vi "Read ECAT VARs.vi"(7 "R/W Case":T7, 8 "error in (no error)":errorcluster, 9 "Output FIFO buffer in":dbl[](array[numeric]), 10 "I/O Input Data in":T1 {"BD Refs"."Data Reference" format="%.0x"}, 11 "I/O Output Vars in":T4[](array[typedef]) {"VS ref" format="%.0x"}) -> (0 "error out":errorcluster, 1 "Output FIFO buffer out":dbl[](array[numeric]), 2 "I/O Input Data out":T1 {"BD Refs"."Data Reference" format="%.0x"}, 3 "I/O Output Vars out":T4[](array[typedef]) {"VS ref" format="%.0x"})   [LabVIEW 2020, in "SEECD Engine.lvlib"]
uses:
  SEECD Engine.lvlib
  Type Defs/RW Case.ctl
  Type Defs/Generic ECAT Slave IOV Cluster.ctl
  <vilib>/NI VeriStand/Custom Device API/Custom Device Item Ref.ctl
  Shared/Type Defs/UDV Data Type.ctl
  Type Defs/Input Data.ctl
  <vilib>/NI VeriStand/Custom Device API/Block Data Reference.ctl
  <vilib>/NI VeriStand/Custom Device API/Data Reference.ctl
  <vilib>/NI VeriStand/Custom Device API/Global Data Refs.vi
  <vilib>/NI VeriStand/Custom Device API/Custom Device API.lvlib
  <vilib>/NI VeriStand/Custom Device Tools/Custom Device Utility Library/Custom Device Utility Library.lvlib
  Shared/SEECD Shared.lvlib
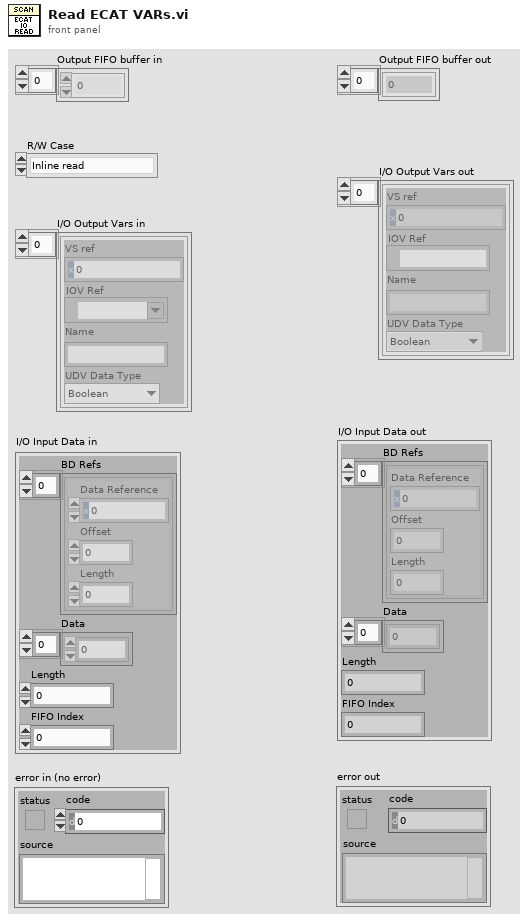
[diagram p1: front panel]
types:
  T1 = typedef "SEECD Engine.lvlib/Input Data.ctl" = cluster{"BD Refs":T2[], "Data":dbl[], "Length":i32, "FIFO Index":i32}
  T2 = typedef "Custom Device API.lvlib/Block Data Reference.ctl" = cluster{"Data Reference":T3, "Offset":u64, "Length":u64}
  T3 = typedef "Custom Device API.lvlib/Data Reference.ctl" = i32
  T4 = typedef "SEECD Engine.lvlib/Generic ECAT Slave IOV Cluster.ctl" = cluster{"VS ref":T5, "IOV Ref":refnum<k21>, "Name":string, "UDV Data Type":T6}
  T5 = typedef "Custom Device API.lvlib/Custom Device Item Ref.ctl" = u64
  T6 = typedef "SEECD Shared.lvlib/UDV Data Type.ctl" = enum16{"Boolean", "Fixed Point", "Int8", "Int16", "Int32", "Int64", "U32 Bit Field", "UInt8", "UInt16", "UInt32", "UInt64", "Other", "DBL", "SGL"}
  T7 = typedef "SEECD Engine.lvlib/RW Case.ctl" = enum16{"Inline read", "Inline write", "Async - Inline loop read", "Async - Inline loop write", "Async loop (read/write)"}
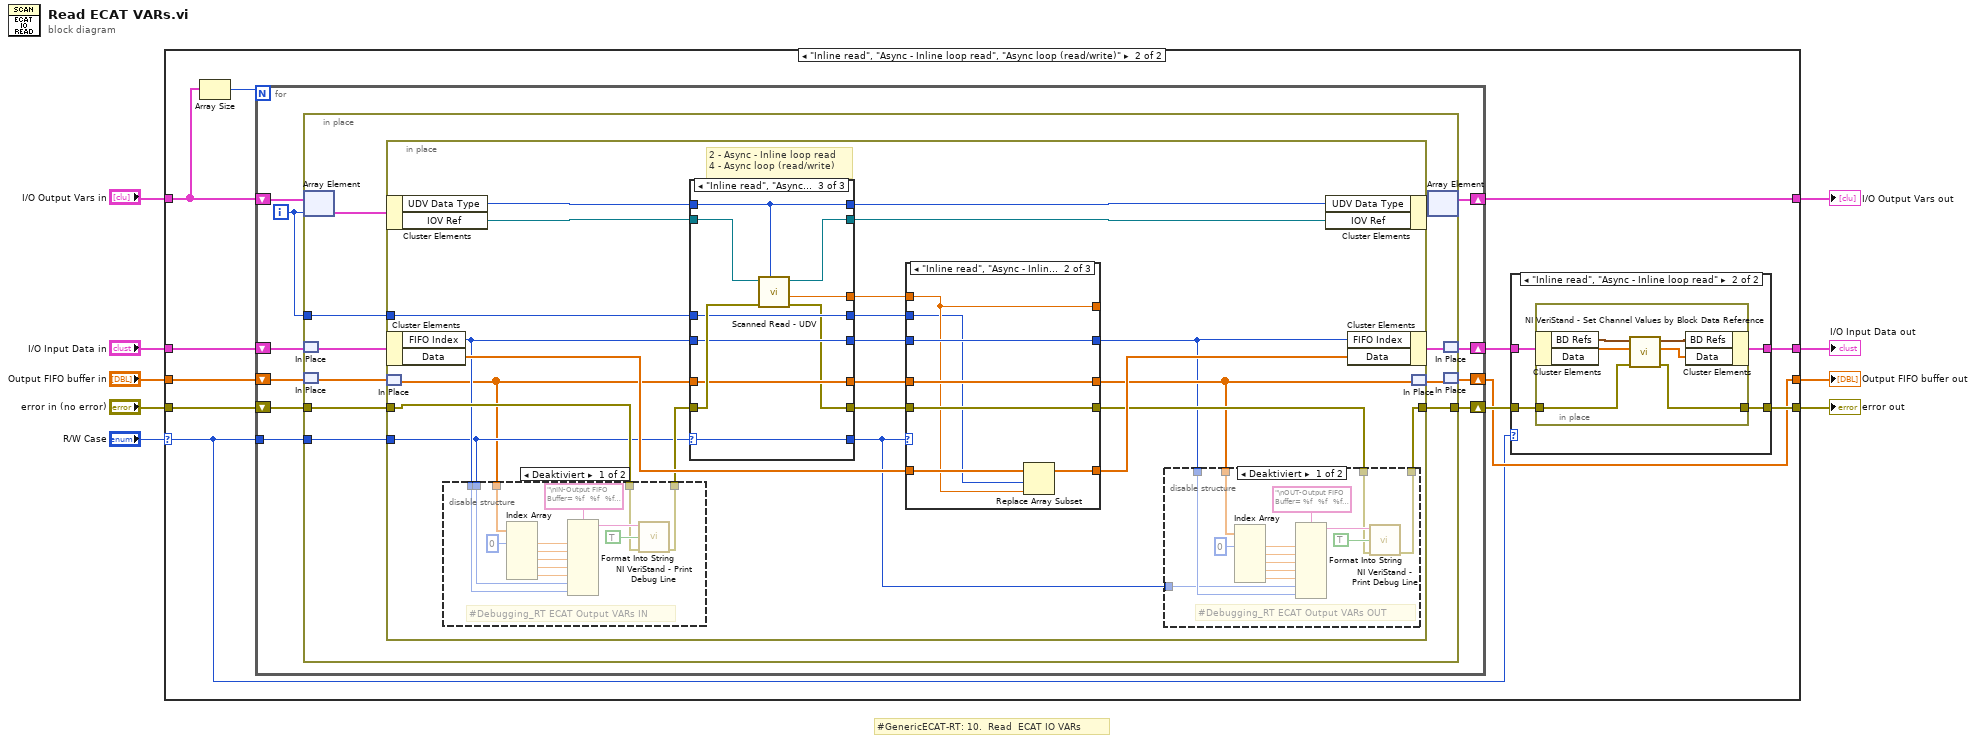
[diagram p0: block diagram]
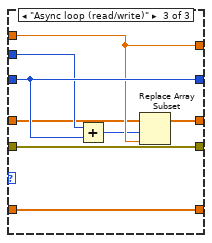
[diagram p7: hidden frame]
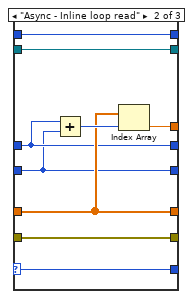
[diagram p9: hidden frame]
diagram:
  # "#GenericECAT-RT: 10.  Read  ECAT IO VARs"
  n1 = case shown="\"Inline read\", \"Async - Inline loop read\", \"Async loop (read/write)\"" "R/W Case" {
    selector: "R/W Case" -> [_ w14]
    tunnel: [w11 w15] -> w9
    tunnel: "Output FIFO buffer in" -> [w11 w25]
    tunnel: [w12 w18] -> w1
    tunnel: [w13 w24] -> w3
    tunnel: "I/O Input Data in" -> [w12 w23]
    tunnel: "I/O Output Vars in" -> [w13 w22]
    tunnel: [w10 w17] -> w7
    tunnel: "error in (no error)" -> [w10 w20]
    frame Default {
    }
    frame "Inline read", "Async - Inline loop read", "Async loop (read/write)" {
      n2 = Array Size(array=w22) -> (size(s)=w21:i32)
      n3 = for {
        N: w21 -> [_]
        shift-right: [w46] -> w24
        shift-left: w22 -> [w47]
        shift-right: [w38] -> w16
        shift-left: w23 -> [w41]
        shift-right: [w44] -> w15
        shift-left: w25 -> [w45]
        shift-right: [w42] -> w19
        shift-left: w20 -> [w43]
        tunnel: w14 -> [w40]
        i -> [w39]
        n4 = in-place {
          in-place-border: w43 -> [w54]
          in-place-border: [w48] -> w42
          in-place-border: w40 -> [w53]
          in-place-border: w39 -> [w52]
          n5 = in-place-array #1(w47, w39) -> (w57:T4)
          n6 = in-place-match #2(w41) -> (w56:T1)
          n7 = in-place-match #3(w45) -> (w55:dbl[])
          n8 = in-place {
            in-place-border: w54 -> [w67]
            in-place-border: w53 -> [w64]
            in-place-border: w52 -> [w76]
            in-place-border: [w61] -> w48
            # "2 - Async - Inline loop read\n4 - Async loop (read/write)"
            n9 = in-place-cluster #4(w57) -> ("UDV Data Type"=w78:T6, "IOV Ref"=w77:refnum<k21>)
            n10 = in-place-cluster #5(w56) -> ("FIFO Index"=w65:i32, "Data"=w79:dbl[])
            n11 = in-place-match #6(w55) -> (w63:dbl[])
            n12 = disable-structure shown="Deaktiviert" {
              disable-tunnel: w67 -> [w99 w109]
              disable-tunnel: [w98 w109] -> w66
              disable-tunnel: w65 -> [w97 _]
              disable-tunnel: w64 -> [w96 _]
              disable-tunnel: w63 -> [w95 _]
              frame Disabled {
                # "#Debugging_RT ECAT Output VARs IN"
                n13 = Index Array(array=w95, index #1=0) -> (element #1=w103:dbl, element #2=w102:dbl, element #3=w101:dbl, element #4=w100:dbl, element #5=w108:dbl)  [unwired: 4 in]
                n14 = Format Into String(format string="\nIN-Output FIFO Buffer= %f   %f   %f   %f   %f   - MODE: %d  - Index: %d\n" ("Format-String"), w103, w102, w101, w100, w108, w96, w97) -> (resulting string=w106:string)  [unwired: 2 in, 1 out]
                n15 = call <vilib>:"NI VeriStand - Print Debug Line.vi"("error in (no error)"=w99, "Add to log file? (F)"=TRUE, "Message"=w106) -> ("error out"=w98:errorcluster)  [unwired: 8 in]
              }
              frame Enabled {
              }
            }
            n16 = case shown="\"Inline read\", \"Async loop (read/write)\"" w64 {
              selector: w64 -> [w130 w140 w147]
              tunnel: w78 -> [w131 w138 w148]
              tunnel: w77 -> [w132 w139 w155]
              tunnel: w65 -> [w134 w141 w151]
              tunnel: w63 -> [w135 w144 w150]
              tunnel: [w135 w144 w150] -> w72
              tunnel: w76 -> [w133 w142 w152]
              tunnel: [_ w143 w146] -> w70
              tunnel: [w133 w142 w152] -> w74
              tunnel: [w134 w141 w151] -> w73
              tunnel: [w130 w140 w147] -> w58
              tunnel: [w132 w139 w154] -> w69
              tunnel: [w131 w138 w148] -> w75
              tunnel: w66 -> [w136 w137 w153]
              tunnel: [w136 w137 w149] -> w71
              frame Default {
              }
              frame "Async - Inline loop read" {
                n17 = Add(x=w142, y=w141) -> (x+y=w145:i32)
                n18 = Index Array(array=w144, index=w145) -> (element=w143:dbl)
              }
              frame "Inline read", "Async loop (read/write)" {
                n19 = call "Scanned Read - UDV.vi"("UDV Data Type"=w148, "error in (no error)"=w153, "IOV ref in"=w155) -> ("error out"=w149:errorcluster, "data out"=w146:dbl, "IOV ref out"=w154:refnum<k21>)  [unwired: 6 in]
              }
            }
            n20 = case shown="\"Inline read\", \"Async - Inline loop read\"" w58 {
              tunnel: w74 -> [_ w115 w125]
              tunnel: w73 -> [w110 w117 w126]
              tunnel: w70 -> [w111 w116 w124]
              tunnel: w72 -> [w112 w118 w123]
              tunnel: w71 -> [w113 w119 w128]
              tunnel: w79 -> [w114 w121 w127]
              tunnel: [w110 w117 w126] -> w59
              tunnel: [w114 w120 w127] -> w68
              tunnel: [w113 w119 w128] -> w62
              tunnel: [w112 w118 w129] -> w60
              tunnel: [w111 w116 w124] -> _
              frame Default {
              }
              frame "Inline read", "Async - Inline loop read" {
                n21 = Replace Array Subset(array=w121, new element=w116, index=w115) -> (w120:dbl[])
              }
              frame "Async loop (read/write)" {
                n22 = Add(x=w125, y=w126) -> (x+y=w122:i32)
                n23 = Replace Array Subset(array=w123, new element=w124, index=w122) -> (w129:dbl[])
              }
            }
            n24 = disable-structure shown="Deaktiviert" {
              disable-tunnel: w62 -> [w84 w94]
              disable-tunnel: [w83 w94] -> w61
              disable-tunnel: w60 -> [w82 _]
              disable-tunnel: w59 -> [w81 _]
              disable-tunnel: w58 -> [w80 _]
              frame Disabled {
                # "#Debugging_RT ECAT Output VARs OUT"
                n25 = Index Array(array=w82, index #1=0) -> (element #1=w88:dbl, element #2=w87:dbl, element #3=w86:dbl, element #4=w85:dbl, element #5=w93:dbl)  [unwired: 4 in]
                n26 = Format Into String(format string="\nOUT-Output FIFO Buffer= %f   %f   %f   %f   %f   - MODE: %d  - Index: %d\n" ("Format-String"), w88, w87, w86, w85, w93, w80, w81) -> (resulting string=w91:string)  [unwired: 2 in, 1 out]
                n27 = call <vilib>:"NI VeriStand - Print Debug Line.vi"("error in (no error)"=w84, "Add to log file? (F)"=TRUE, "Message"=w91) -> ("error out"=w83:errorcluster)  [unwired: 8 in]
              }
              frame Enabled {
              }
            }
            n28 = in-place-cluster #4("UDV Data Type"=w75, "IOV Ref"=w69) -> (w51:T4)
            n29 = in-place-cluster #5("FIFO Index"=w59, "Data"=w68) -> (w50:T1)
            n30 = in-place-match #6(w60) -> (w49:dbl[])
          }
          n31 = in-place-array #1(w51) -> (w46:T4[])  [unwired: 1 out]
          n32 = in-place-match #2(w50) -> (w38:T1)
          n33 = in-place-match #3(w49) -> (w44:dbl[])
        }
      }
      n34 = case shown="\"Inline read\", \"Async - Inline loop read\"" w14 {
        tunnel: w16 -> [w26 w28]
        tunnel: w19 -> [w27 w31]
        tunnel: [w27 w30] -> w17
        tunnel: [w26 w29] -> w18
        frame Default {
        }
        frame "Inline read", "Async - Inline loop read" {
          n35 = in-place {
            in-place-border: w31 -> [w35]
            in-place-border: [w34] -> w30
            n36 = in-place-cluster #7(w28) -> ("BD Refs"=w32:T2[], "Data"=w33:dbl[])
            n37 = call <vilib>:"NI VeriStand - Set Channel Values by Block Data Reference.vi"("error in (no error)"=w35, "Values Array in"=w33, "Block Data Ref"=w32) -> ("error out"=w34:errorcluster, "Values Array out"=w36:dbl[], "Block Data Ref dup"=w37:T2[])  [unwired: 6 in]
            n38 = in-place-cluster #7("BD Refs"=w37, "Data"=w36) -> (w29:T1)
          }
        }
      }
    }
  }
  "Output FIFO buffer out" <- w9
  "error out" <- w7
  "I/O Output Vars out" <- w3
  "I/O Input Data out" <- w1
